vi "Init.vi"(6 "Column Definitions":T9[](array[typedef]) {"MinWidth" min=2 step=1; "AutoSizeMode" items=["None"=1, "ColumnHeader"=2, "AllCellsExceptHeader"=4, "AllCells"=6, "DisplayedCellsExceptHeader"=8, "DisplayedCells"=10, "Fill"=16]; "FillWeight" min=1 max=100}, 8 "error in (no error)":errorcluster, 9 "object refs":T8, 10 "References in":T1, 11 "Multi Column Listbox in":refnum<class "Multi Column Listbox.lvclass">) -> (0 "error out":errorcluster, 2 "Registered Events":refnum<event-registration>, 3 "Multi Column Listbox out":refnum<class "Multi Column Listbox.lvclass">)   [LabVIEW 2013, in "Table Manager.lvlib" / "Multi Column Listbox.lvclass"]
uses:
  Multi Column Listbox.lvclass
  LabVIEWdotNetDataGrid/source/Events/Abstract EVENT/Abstract EVENT.lvclass
  Column/Column Descriptor.ctl
  Column/Column Type.ctl
  <vilib>/NI/Tag Bus/tag/Data Type.ctl
  TagSelectModule/Source/editor node/object ref.ctl
  TagSelectModule/Source/editor node/tag select module editor node.lvclass
  <vilib>/NI/Tag Bus Data Framework/Configuration Editor/Classes/Engine Parent/Engine Parent Editor Node.lvclass
  TagSelectModule/Source/editor node/references.ctl
  <vilib>/NI/Configuration Framework/Node/StopEvent.ctl
  <vilib>/NI/Configuration Framework/Node/RefreshUIEvent.ctl
  <vilib>/NI/Configuration Framework/Node/CacheState.ctl
  <vilib>/NI/Configuration Framework/Node/NodeChangeEvent.ctl
  <vilib>/NI/Configuration Framework/Node/NodeRef.ctl
  <vilib>/NI/Configuration Framework/Node/NISE_CEF_Node.lvclass
  <vilib>/NI/Tag Bus Data Framework/control module/editor node/channel action event.ctl
  <vilib>/NI/Tag Bus Data Framework/control module/editor node/dialog output action.ctl
  <vilib>/NI/Tag Bus Module Framework/channel/TBM channel.lvclass
  <vilib>/NI/Tag Bus/tag/tag descriptor.lvclass
  <vilib>/NI/AMC/Message Queue.ctl
  <vilib>/NI/AMC/Message.ctl
  <vilib>/NI/Tools/Keyed Array/KeyedArray.ctl
  <vilib>/NI/Configuration Framework/Node/UserEventRef.ctl
  <vilib>/NI/Configuration Framework/Controls/EventCluster.ctl
  Line/Line.lvclass
  Table Manager/Table Manager.lvclass/Table Manager.ctl
  Multi Column Listbox.lvclass/Multi Column Listbox.ctl
  String Column/String Column.lvclass
  Column/Column.lvclass/Column.ctl
  Listbox Enum Column/List Box Enum Column.lvclass
  Listbox Enum Column/List Box Enum Column.lvclass/List Box Enum Column.ctl
  Tag Channel Column/Tag Channel Column.lvclass
  Tag Channel Column/Tag Channel Column.lvclass/Tag Channel Column.ctl
  Line/Line.lvclass/Line.ctl
  Column/Write Header.vi
  Listbox Enum Column/Write Enum Reference.vi
  Tag Channel Column/Write Channel suffix.vi
  Table Manager/Write ATM.vi
  Read Listbox.vi
  Line/Write Line UID.vi
  Line/Write Columns.vi
  Table Manager/Write Line.vi
  Column/Column.lvclass
  <vilib>/NI/Tag Bus Data Framework/control module/editor node/control module editor.lvclass
  <vilib>/NI/Tools/Keyed Array/Tools_KeyedArray.lvlib
  <vilib>/NI/AMC/AMC.lvlib
  <vilib>/NI/Configuration Framework/NISE_CEF_TreeControl.lvlib
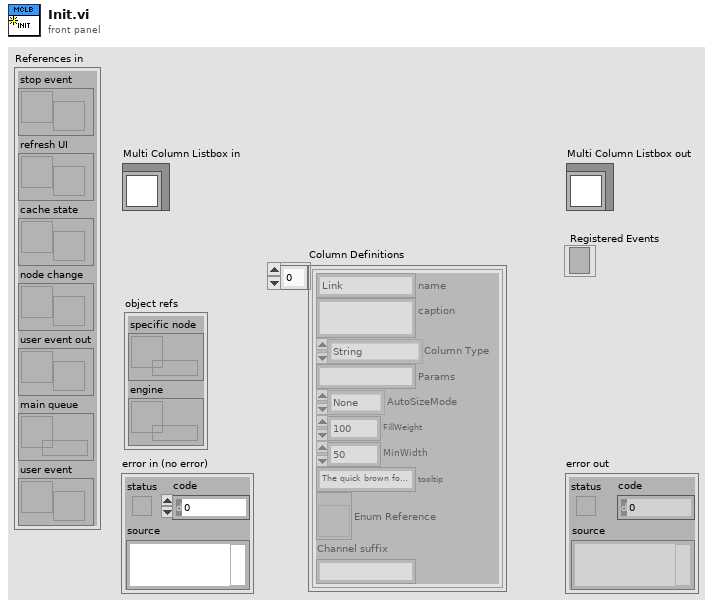
[diagram p1: front panel]
types:
  T1 = typedef "tag select module editor node.lvclass/references.ctl" = cluster{"stop event":T2, "refresh UI":T3, "cache state":T4, "node change":T5, "user event out":refnum<user-event>, "main queue":T6, "user event":T7}
  T2 = typedef "NISE_CEF_Node.lvclass/StopEvent.ctl" = refnum<user-event>
  T3 = typedef "NISE_CEF_Node.lvclass/RefreshUIEvent.ctl" = refnum<user-event>
  T4 = typedef "NISE_CEF_Node.lvclass/CacheState.ctl" = refnum<user-event>
  T5 = typedef "NISE_CEF_Node.lvclass/NodeChangeEvent.ctl" = refnum<user-event>
  T6 = typedef "AMC.lvlib/Message Queue.ctl" = refnum<queue>
  T7 = typedef "NISE_CEF_Node.lvclass/UserEventRef.ctl" = refnum<user-event>
  T8 = typedef "tag select module editor node.lvclass/object ref.ctl" = cluster{"specific node":refnum<data-value>, "engine":refnum<data-value>}
  T9 = typedef "Table Manager.lvlib/Column.lvclass/Column Descriptor.ctl" = cluster{"name":string, "caption":string, "Column Type":T10, "Params":string, "AutoSizeMode":i32, "FillWeight":sgl, "MinWidth":u32, "tooltip":string, "Enum Reference":refnum<vi>, "Channel suffix":string}
  T10 = typedef "Table Manager.lvlib/Column.lvclass/Column Type.ctl" = enum16{"String", "Enum", "Tag", "Numeric"}
  T11 = typedef "control module editor.lvclass/channel action event.ctl" = cluster{"action":T12, "channel":refnum<class "TBM channel.lvclass">, "selected tag":refnum<class "tag descriptor.lvclass">}
  T12 = typedef "control module editor.lvclass/dialog output action.ctl" = enum16{"Tag Created", "Tag Selected", "Set Default", "disconnect"}
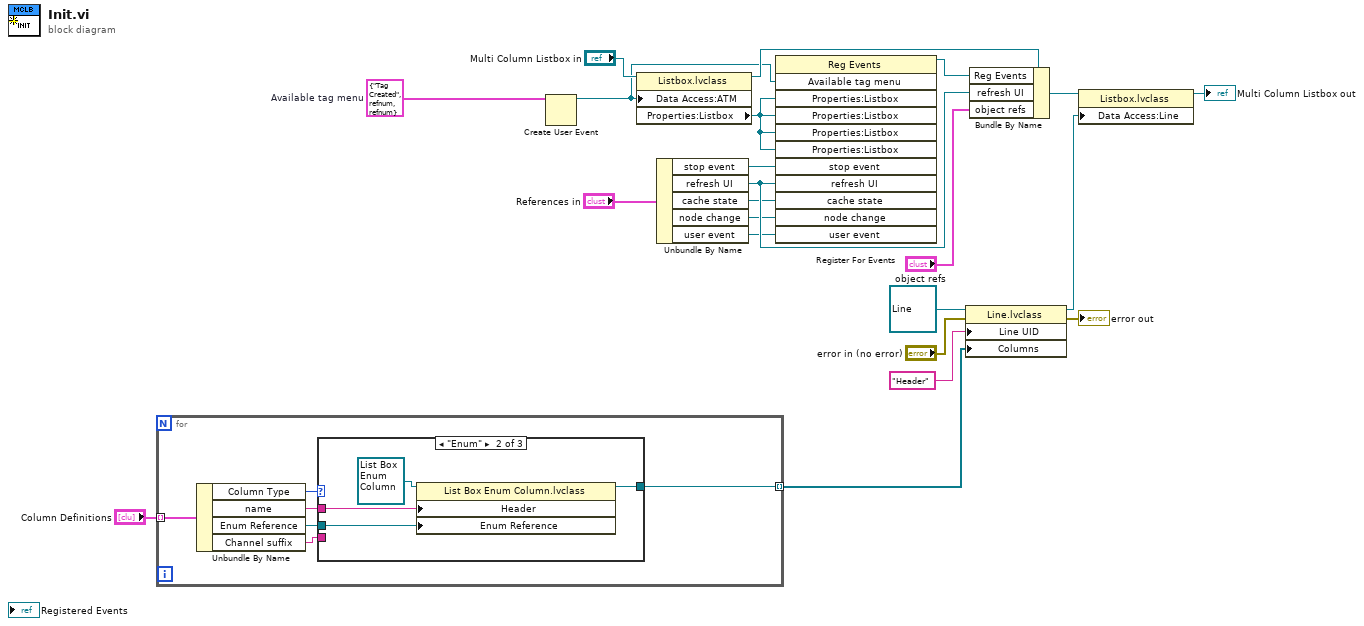
[diagram p0: block diagram]
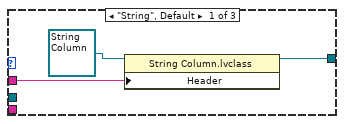
[diagram p2: hidden frame]
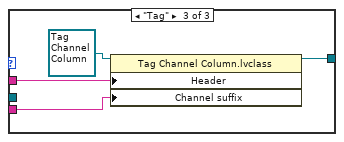
[diagram p3: hidden frame]
diagram:
  w10 = T11 {"action"=enum."Tag Created", "channel"=refnum, "selected tag"=refnum}  # Available tag menu
  n1 = for {
    tunnel: "Column Definitions" -> [w28] mode=indexing
    tunnel: [w26] -> w19 mode=indexing
    n2 = Unbundle By Name(w28) -> ("Column Type"=w27:T10, "name"=w25:string, "Enum Reference"=w24:refnum<vi>, "Channel suffix"=w23:string)
    n3 = case shown="\"Enum\"" w27 {
      tunnel: [w29 w34 w38] -> w26
      tunnel: w25 -> [w30 w33 w37]
      tunnel: w24 -> [_ w32 _]
      tunnel: w23 -> [_ _ w36]
      frame "String", Default {
        n4 = property class="String Column.lvclass"(reference=refnum<class "String Column.lvclass"> refnum ("Table Manager.lvlib:String Column.lvclass"), "Header"=w30) -> (reference out=w29:refnum<class "String Column.lvclass">)  [unwired: 1 in, 1 out]
      }
      frame "Enum" {
        n5 = property class="List Box Enum Column.lvclass"(reference=refnum<class "List Box Enum Column.lvclass"> refnum ("Table Manager.lvlib:List Box Enum Column.lvclass"), "Header"=w33, "Enum Reference"=w32) -> (reference out=w34:refnum<class "List Box Enum Column.lvclass">)  [unwired: 1 in, 1 out]
      }
      frame "Tag" {
        n6 = property class="Tag Channel Column.lvclass"(reference=refnum<class "Tag Channel Column.lvclass"> refnum ("Table Manager.lvlib:Tag Channel Column.lvclass"), "Header"=w37, "Channel suffix"=w36) -> (reference out=w38:refnum<class "Tag Channel Column.lvclass">)  [unwired: 1 in, 1 out]
      }
    }
  }
  n7 = Create User Event(user event datatype=w10) -> (user event=w9:refnum<user-event>)  [unwired: 1 in, 1 out]
  n8 = property class="Listbox.lvclass"(reference="Multi Column Listbox in", "Data Access:ATM"=w9) -> (reference out=w14:refnum<class "Multi Column Listbox.lvclass">, "Properties:Listbox"=w12:refnum<vi>)  [unwired: 1 in, 1 out]
  n9 = Unbundle By Name("References in") -> ("stop event"=w7:T2, "refresh UI"=w6:T3, "cache state"=w5:T4, "node change"=w4:T5, "user event"=w3:T7)
  n10 = register-events(w9, w12, w12, w12, w12, w7, w6, w5, w4, w3) -> (reference out=w2:refnum<event-registration>)  [unwired: 2 in, 1 out]
  n11 = property class="Line.lvclass"(reference=refnum<class "Line.lvclass"> refnum ("Table Manager.lvlib:Line.lvclass"), error in="error in (no error)", "Line UID"="Header", "Columns"=w19) -> (reference out=w16:refnum<class "Line.lvclass">, error out=→"error out":errorcluster)
  n12 = Bundle By Name(cluster=w14, "Reg Events"=w2, "refresh UI"=w6, "object refs"="object refs") -> (w13:refnum<class "Multi Column Listbox.lvclass">)
  n13 = property class="Listbox.lvclass"(reference=w13, "Data Access:Line"=w16) -> (reference out=→"Multi Column Listbox out":refnum<class "Multi Column Listbox.lvclass">)  [unwired: 1 in, 1 out]
